vi "test Read And Write Anchor.vi"(8 "error in (no error)":errorcluster, 11 "TestCase in":refnum<class "AnchorTests.lvclass">) -> (0 "error out":errorcluster, 3 "TestCase out":refnum<class "AnchorTests.lvclass">)   [LabVIEW 2014, in "AnchorTests.lvclass"]
uses:
  AnchorTests.lvclass
  <vilib>/addons/_JKI Toolkits/VI Tester/TestCase.llb/TestCase.lvclass
  SPLAT/Anchor/Anchor.lvclass
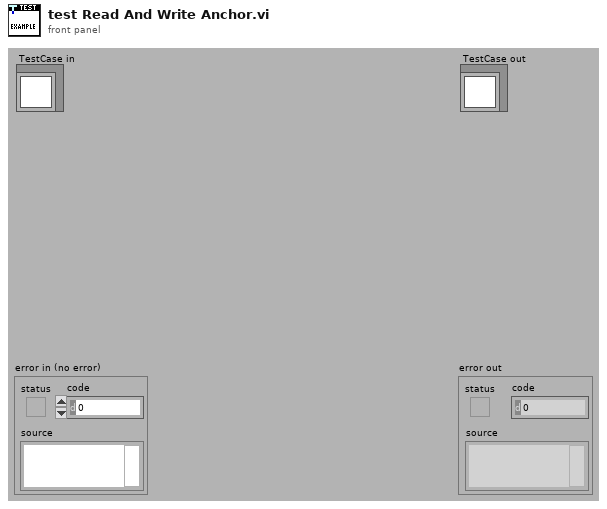
[diagram p1: front panel]
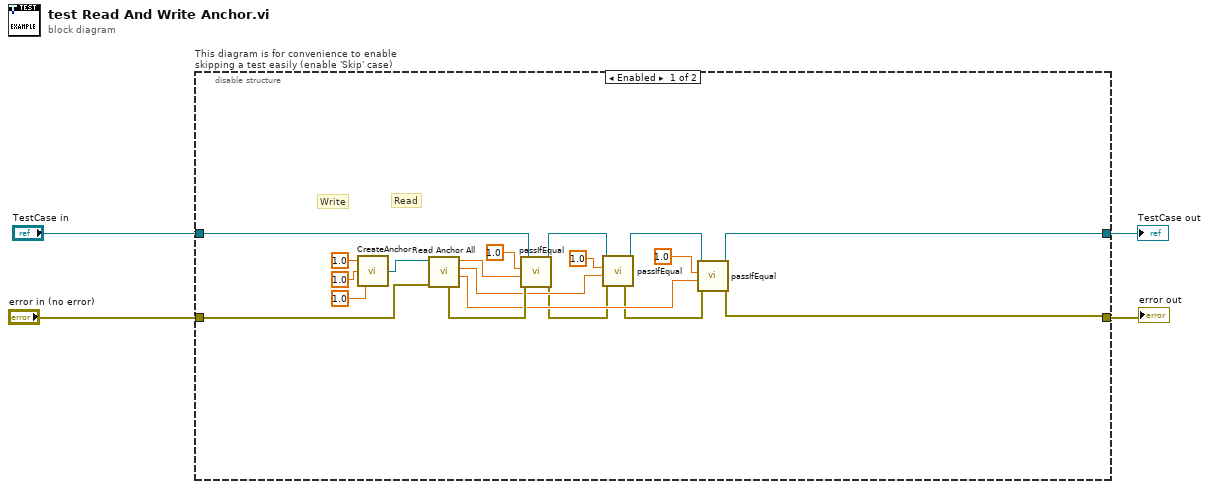
[diagram p0: block diagram]
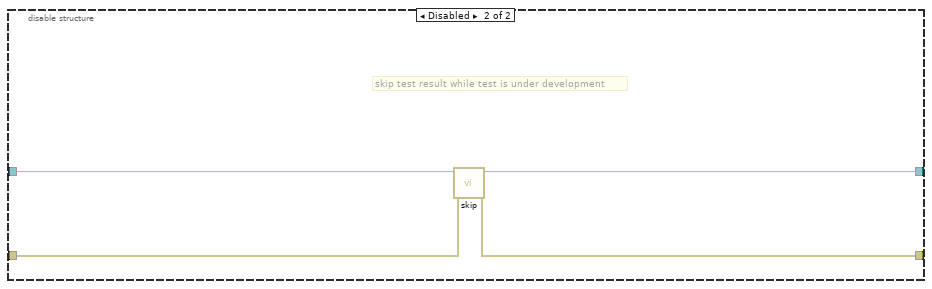
[diagram p2: hidden frame]
diagram:
  n1 = disable-structure "This diagram is for convenience to enable skipping a test easily (enable 'Skip' case)" shown="Enabled" {
    disable-tunnel: "TestCase in" -> [w16 w27]
    disable-tunnel: [w23 w25] -> w1
    disable-tunnel: [w22 w26] -> w3
    disable-tunnel: "error in (no error)" -> [w17 w24]
    frame Enabled {
      # "Read"
      # "Write"
      n2 = call "CreateAnchor.vi"("Anchor Y"=1.0, "Anchor X"=1.0, "Anchor ID"=1.0) -> ("Anchor Out"=w18:refnum<class "Anchor.lvclass">)
      n3 = call "Read Anchor All.vi"("error in (no error)"=w17, "Anchor in"=w18) -> ("AnchorY"=w7:dbl, "AnchorX"=w8:dbl, "AnchorID"=w12:dbl, "error out"=w11:errorcluster)  [unwired: 4 in, 2 out]
      n4 = call-dynamic "passIfEqual.vi"("error in (no error)"=w11, "y"=w12, "x"=1.0 ("Anchor ID"), "TestCase in"=w16) -> ("error out"=w6:errorcluster, "TestCase out"=w15:refnum<class "AnchorTests.lvclass">)  [unwired: 6 in]
      n5 = call-dynamic "passIfEqual.vi"("error in (no error)"=w6, "y"=w8, "x"=1.0 ("Anchor ID"), "TestCase in"=w15) -> ("error out"=w5:errorcluster, "TestCase out"=w14:refnum<class "AnchorTests.lvclass">)  [unwired: 6 in]
      n6 = call-dynamic "passIfEqual.vi"("error in (no error)"=w5, "y"=w7, "x"=1.0 ("Anchor ID"), "TestCase in"=w14) -> ("error out"=w22:errorcluster, "TestCase out"=w23:refnum<class "AnchorTests.lvclass">)  [unwired: 6 in]
    }
    frame Disabled {
      # "skip test result while test is under development"
      n7 = call <vilib>:"skip.vi"("error in (no error)"=w24, "TestCase in"=w27) -> ("error out"=w26:errorcluster, "TestCase out"=w25:refnum<class "AnchorTests.lvclass">)  [unwired: 8 in]
    }
  }
  "error out" <- w3
  "TestCase out" <- w1
